vi "Sigmoid.vi"(1 "x":dbl) -> (0 "sigmoid(x)":dbl)   [LabVIEW 2025]
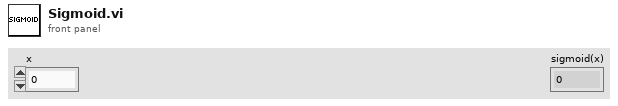
[diagram p1: front panel]
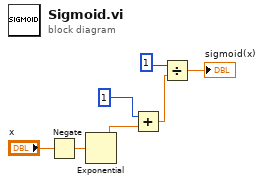
[diagram p0: block diagram]
diagram:
  n1 = Negate(x="x") -> (-x=w6:dbl)
  n2 = Exponential(1:w6) -> (0:w4:dbl)
  n3 = Add(x=1, y=w4) -> (x+y=w2:dbl)
  n4 = Divide(x=1, y=w2) -> (x/y=→"sigmoid(x)":dbl)
